vi "Get Camera Status.vi"(8 "error in (no error)":errorcluster, 11 "CCDCamera in":refnum<class "CCDCamera.lvclass">) -> (0 "error out":errorcluster, 2 "Cluster":T1, 3 "CCDCamera out":refnum<class "CCDCamera.lvclass">)   [LabVIEW 2012, in "CCDCamera.lvclass"]
doc: "This VI returns the CCD dimensions, the serial number, the initialization status, the setted temperature, the current temperature, the last image, and the error in of the class."
uses:
  CCDCamera.lvclass
  CCDCamera.lvclass/CCDCamera.ctl
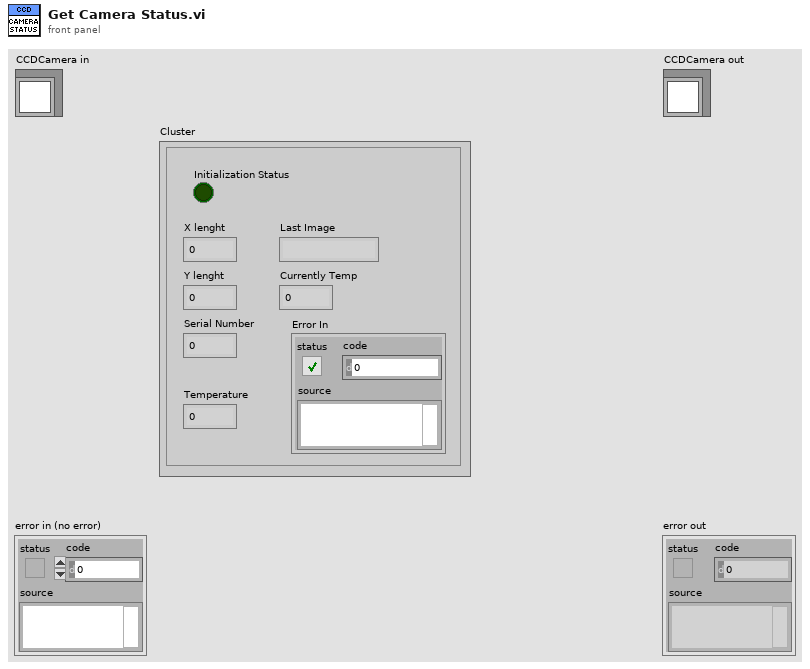
[diagram p1: front panel]
types:
  T1 = cluster{"Initialization Status":bool, "X lenght":dbl, "Y lenght":dbl, "Serial Number":dbl, "Temperature":dbl, "Last Image":string, "Currently Temp":dbl, "Error In":errorcluster}
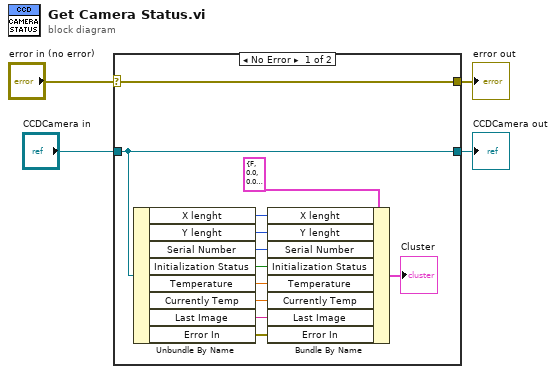
[diagram p0: block diagram]
diagram:
  n1 = case shown="No Error" "error in (no error)" {
    selector: "error in (no error)" -> [w16 w18]
    tunnel: [w16 w18] -> w3
    tunnel: [w15 w17] -> w1
    tunnel: "CCDCamera in" -> [w15 w17]
    frame No Error {
      n2 = Unbundle By Name(w15) -> ("X lenght"=w12:u16, "Y lenght"=w11:u16, "Serial Number"=w10:u16, "Initialization Status"=w9:bool, "Temperature"=w8:dbl, "Currently Temp"=w7:dbl, "Last Image"=w6:string, "Error In"=w5:errorcluster)
      n3 = Bundle By Name(cluster=T1 {"Initialization Status"=FALSE, "X lenght"=0.0, "Y lenght"=0.0, "Serial Number"=0.0, "Temperature"=0.0, "Last Image"="", "Currently Temp"=0.0, "Error In"={"status"=FALSE, "code"=0, "source"=""}} ("Cluster 2"), "X lenght"=w12, "Y lenght"=w11, "Serial Number"=w10, "Initialization Status"=w9, "Temperature"=w8, "Currently Temp"=w7, "Last Image"=w6, "Error In"=w5) -> (→"Cluster":T1)
    }
    frame Error {
    }
  }
  "error out" <- w3
  "CCDCamera out" <- w1
